vi "Router - Initial Handshaking.vi"(8 "error in (no error)":errorcluster, 11 "Router Data In":T1) -> (0 "error out":errorcluster, 3 "Router Data Out":T1)   [LabVIEW 2016, in "PXImc Router.lvlib"]
uses:
  PXImc Router.lvlib
  Controls/Router - Configuration.ctl
  Controls/Router/Node Block R-W Properties.ctl
  Controls/Router/Block Properties.ctl
  Controls/Router/Router - PXImc Properties.ctl
  Controls/Router/Router - PXImc Card Properties.ctl
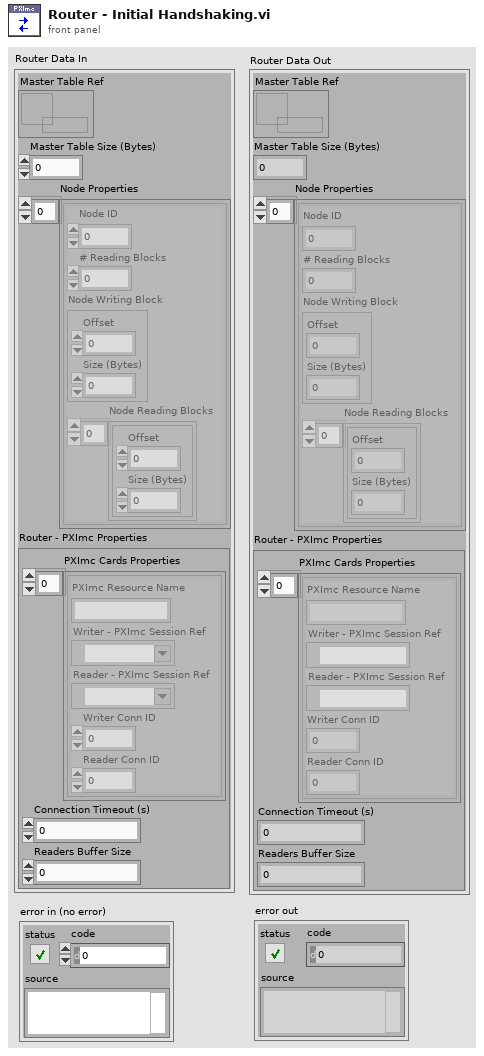
[diagram p1: front panel]
types:
  T1 = typedef "PXImc Router.lvlib/Router - Configuration.ctl" = cluster{"Master Table Ref":refnum<data-value>, "Master Table Size (Bytes)":u32, "Node Properties":T2[], "Router - PXImc Properties":T4}
  T2 = typedef "PXImc Router.lvlib/Node Block R-W Properties.ctl" = cluster{"Node ID":u32, "# Reading Blocks":u32, "Node Writing Block":T3, "Node Reading Blocks":T3[]}
  T3 = typedef "PXImc Router.lvlib/Block Properties.ctl" = cluster{"Offset":u32, "Size (Bytes)":u32}
  T4 = typedef "PXImc Router.lvlib/Router - PXImc Properties.ctl" = cluster{"PXImc Cards Properties":T5[], "Connection Timeout (s)":dbl, "Readers Buffer Size":u64}
  T5 = typedef "PXImc Router.lvlib/Router - PXImc Card Properties.ctl" = cluster{"PXImc Resource Name":string, "Writer - PXImc Session Ref":refnum<k21>, "Reader - PXImc Session Ref":refnum<k21>, "Writer Conn ID":u16, "Reader Conn ID":u16}
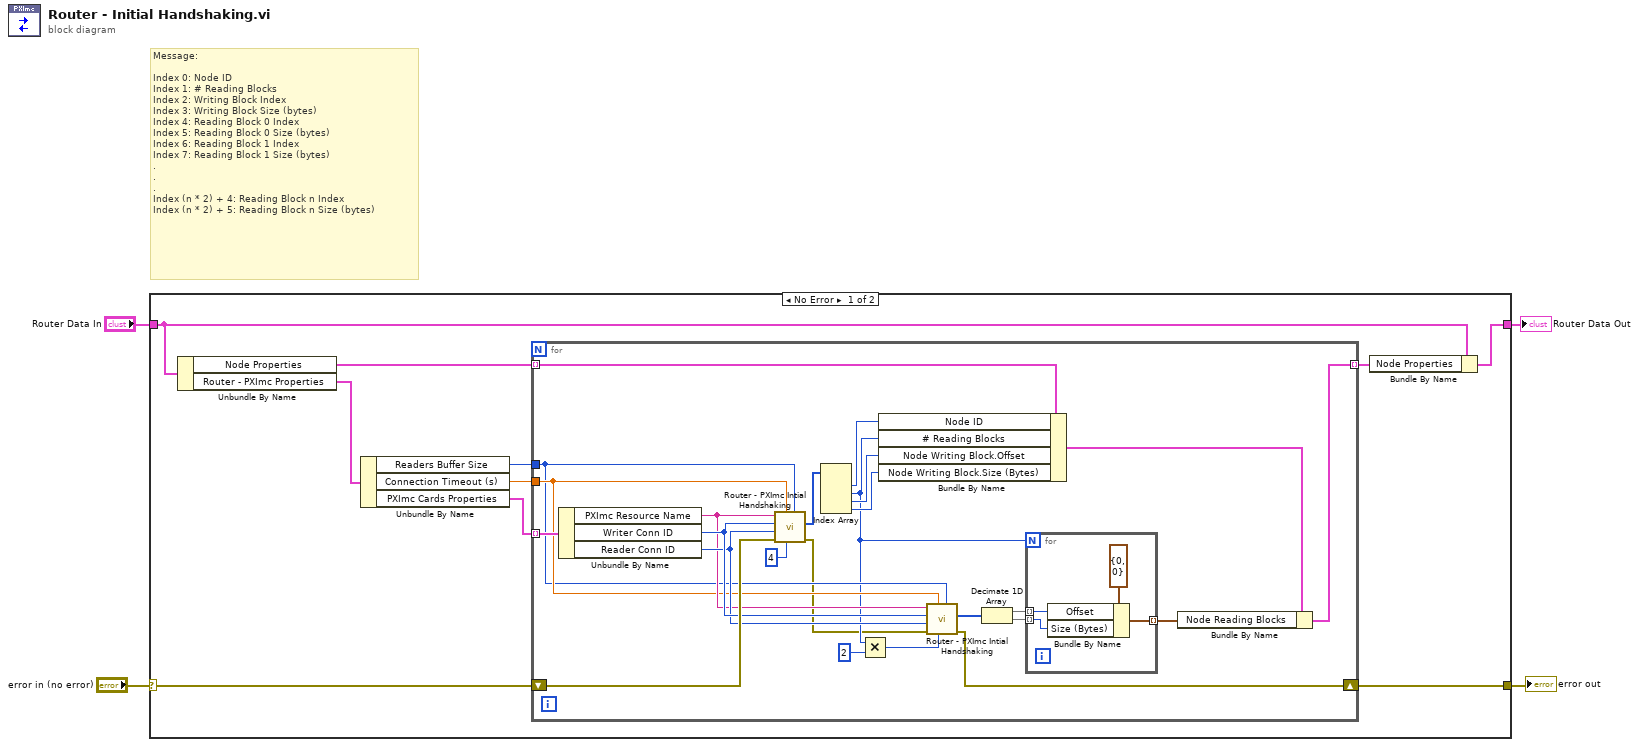
[diagram p0: block diagram]
diagram:
  # "Message:\n\nIndex 0: Node ID\nIndex 1: # Reading Blocks\nIndex 2: Writing Block Index\nIndex 3: Writing Block Size (bytes)\nIndex 4: Reading Block 0 Index\nIndex 5: Reading Block 0 Size (bytes)\nIndex 6: Reading Block 1 Index\nIndex 7: Reading Block 1 Size (bytes)\n.\n.\n.\nIndex (n * 2) + 4: Reading Block n Index\nIndex (n * 2) + 5: Reading Block n Size (bytes)"
  n1 = case shown="No Error" "error in (no error)" {
    selector: "error in (no error)" -> [w14 w44]
    tunnel: [w13 w44] -> w3
    tunnel: "Router Data In" -> [w7 w43]
    tunnel: [w6 w43] -> w1
    frame No Error {
      n2 = Unbundle By Name(w7) -> ("Node Properties"=w9:T2[], "Router - PXImc Properties"=w8:T4)
      n3 = Unbundle By Name(w8) -> ("Readers Buffer Size"=w10:u64, "Connection Timeout (s)"=w11:dbl, "PXImc Cards Properties"=w12:T5[])
      n4 = for {
        shift-right: [w16] -> w13
        shift-left: w14 -> [w31]
        tunnel: w12 -> [w37] mode=indexing
        tunnel: w11 -> [w25]
        tunnel: w10 -> [w24]
        tunnel: w9 -> [w35] mode=indexing
        tunnel: [w15] -> w5 mode=indexing
        n5 = Unbundle By Name(w37) -> ("PXImc Resource Name"=w26:string, "Writer Conn ID"=w28:u16, "Reader Conn ID"=w27:u16)
        n6 = call "Router - PXImc Intial Handshaking.vi"("Reader Buffer Size In"=w24, "# Elements to Read"=4, "Connection Timeout (s)"=w25, "error in (no error)"=w31, "Reader Conn ID"=w27, "Writer Conn ID"=w28, "Resource Name In"=w26) -> ("error out"=w17:errorcluster, "Data Out"=w36:u32[])  [unwired: 3 in]
        n7 = Index Array(array=w36) -> (element #1=w34:u32, element #2=w22:u32, element #3=w33:u32, element #4=w32:u32)  [unwired: 4 in]
        n8 = Multiply(x=w22, y=u32 2) -> (x*y=w29:u32)
        n9 = Bundle By Name(cluster=w35, "Node ID"=w34, "# Reading Blocks"=w22, "Node Writing Block.Offset"=w33, "Node Writing Block.Size (Bytes)"=w32) -> (w23:T2)
        n10 = call "Router - PXImc Intial Handshaking.vi"("Reader Buffer Size In"=w24, "# Elements to Read"=w29, "Connection Timeout (s)"=w25, "error in (no error)"=w17, "Reader Conn ID"=w27, "Writer Conn ID"=w28, "Resource Name In"=w26) -> ("error out"=w16:errorcluster, "Data Out"=w20:u32[])  [unwired: 3 in]
        n11 = Decimate 1D Array(w20) -> (w18:u32[], w19:u32[])
        n12 = for {
          N: w22 -> [_]
          tunnel: [w41] -> w21 mode=indexing
          tunnel: w19 -> [w39] mode=indexing
          tunnel: w18 -> [w40] mode=indexing
          n13 = Bundle By Name(cluster=T3 {"Offset"=0, "Size (Bytes)"=0} ("Node Writing Block"), "Offset"=w40, "Size (Bytes)"=w39) -> (w41:T3)
        }
        n14 = Bundle By Name(cluster=w23, "Node Reading Blocks"=w21) -> (w15:T2)
      }
      n15 = Bundle By Name(cluster=w7, "Node Properties"=w5) -> (w6:T1)
    }
    frame Error {
    }
  }
  "error out" <- w3
  "Router Data Out" <- w1
